vi "00 - DAQmx IO.vi"() -> ()   [LabVIEW 2021]
panel:
  in  "stop (F)":bool
  # "Open Block Diagram to see DAQmx Hardware Connections\nCtl + E (instructions on diagram)"
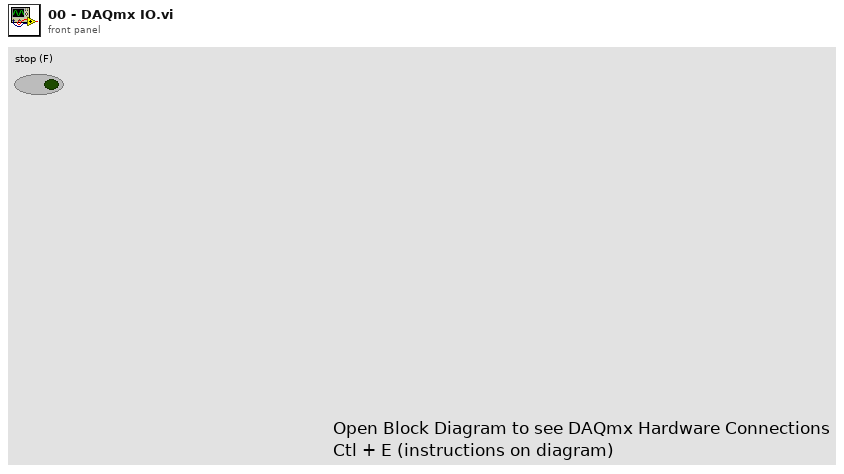
[diagram p1: front panel]
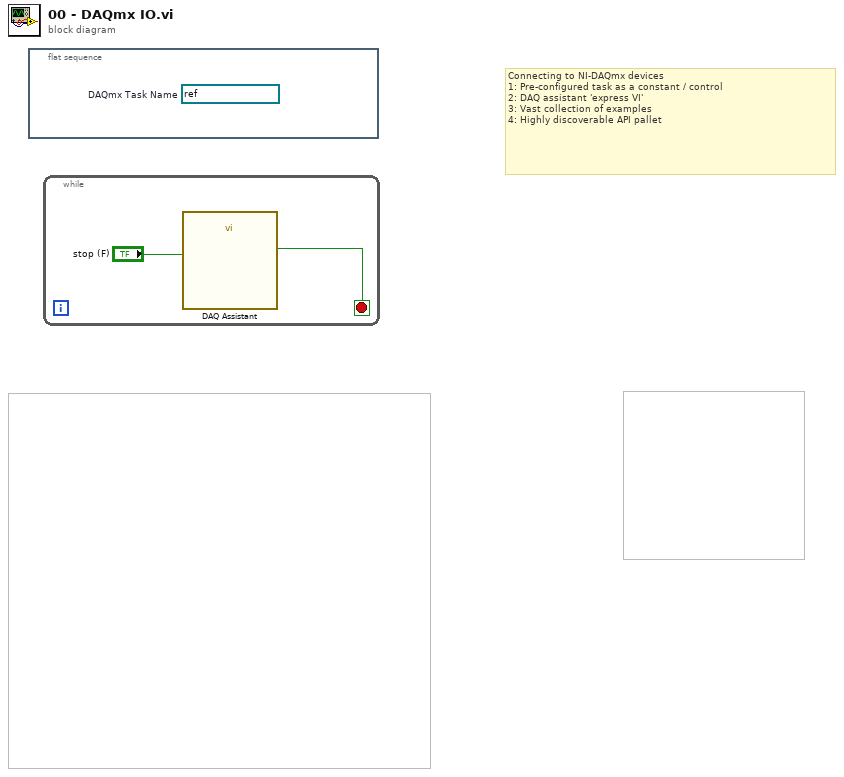
[diagram p0: block diagram]
diagram:
  # "Connecting to NI-DAQmx devices\n1: Pre-configured task as a constant / control\n2: DAQ assistant 'express VI'\n3: Vast collection of examples\n4: Highly discoverable API pallet"
  n1 = flat-sequence {
    frame #0 {
      (unwired) refnum<k21> "MyStrainTask"  # DAQmx Task Name
    }
  }
  n2 = while {
    stop <- w1 stop-if-true
    n3 = call "DAQ Assistant"("stop (F)"="stop (F)") -> ("stopped"=w1:bool)  [unwired: 15 in, 3 out]
  }
